vi "TCP_NODELAY.vi"(8 "error in (no error)":errorcluster, 10 "Disable Nagle":bool, 11 "Network Connection in":refnum<k5>) -> (0 "error out":errorcluster, 3 "Network Connection out":refnum<k5>)   [LabVIEW 2013, in "Modbus Library - Advance.lvlib"]
doc: "This VI disables the nagle algorithm on a port."
uses:
  Modbus Library - Advance.lvlib
  wsock32.dll
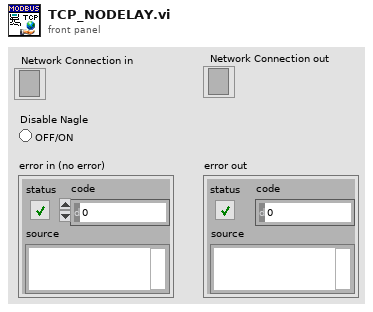
[diagram p1: front panel]
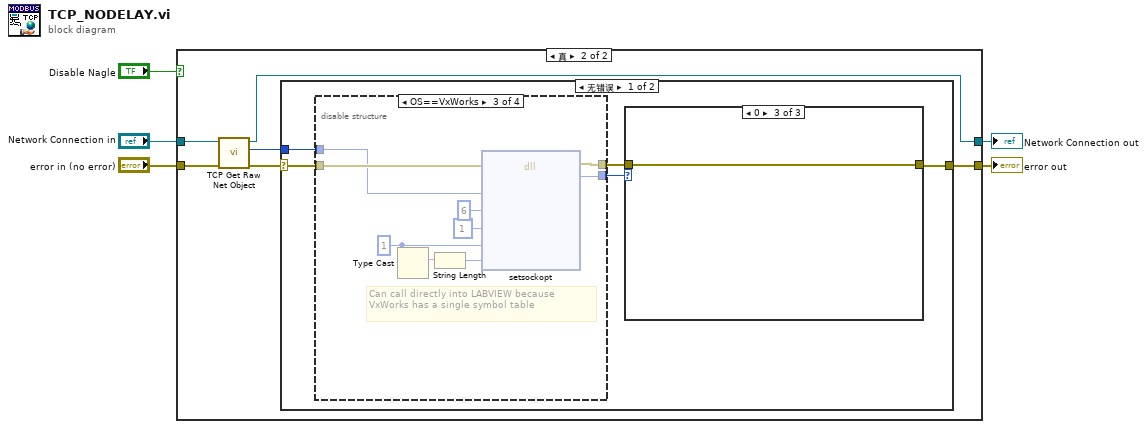
[diagram p0: block diagram]
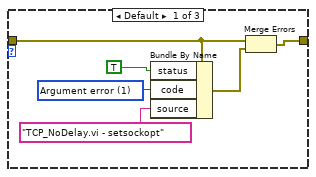
[diagram p3: hidden frame]
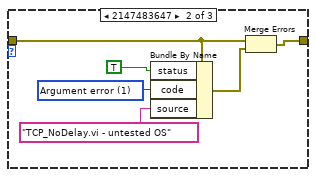
[diagram p4: hidden frame]
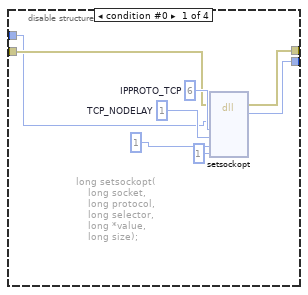
[diagram p5: hidden frame]
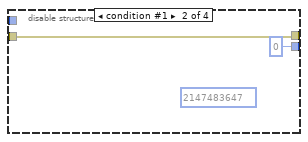
[diagram p6: hidden frame]
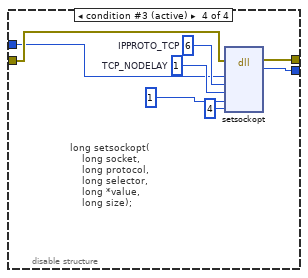
[diagram p7: hidden frame]
diagram:
  n1 = case shown="真" "Disable Nagle" {
    tunnel: "Network Connection in" -> [w7 w13]
    tunnel: [w7 w12] -> w1
    tunnel: "error in (no error)" -> [w6 w11]
    tunnel: [w6 w9] -> w2
    frame False {
    }
    frame True {
      n2 = call <vilib>:"TCP Get Raw Net Object.vi"("error in (no error)"=w11, "connection ID"=w13) -> ("error out"=w10:errorcluster, "raw net object"=w8:u64, "connection ID out"=w12:refnum<k5>)  [unwired: 7 in]
      n3 = case shown="无错误" w10 {
        selector: w10 -> [w18 w59]
        tunnel: [w14 w59] -> w9
        tunnel: w8 -> [w17 _]
        frame No Error {
          n4 = disable-structure shown="OS==VxWorks" {
            disable-tunnel: w18 -> [w36 w41 w45 w52]
            disable-tunnel: w17 -> [w34 _ w42 w51]
            disable-tunnel: [w33 w41 w44 w55] -> w15
            disable-tunnel: [w32 0 w43 w54] -> w16
            frame condition #0 {
              w38 = 1  # TCP_NODELAY
              w37 = 6  # IPPROTO_TCP
              # "long setsockopt(\n    long socket,\n    long protocol,\n    long selector,\n    long *value,\n    long size);"
              n5 = dll-call lib="wsock32.dll" fn="setsockopt" ("Call Library Function")(error in=w36, "socket"=w34, "protocol"=w37, "selector"=w38, "value"=u8 1, "size"=1) -> (error out=w33:errorcluster, w32:i32)  [unwired: 7 in, 1 out]
            }
            frame condition #1 {
              (unwired) 2147483647
            }
            frame condition #2 {
              w48 = 1 ("(char*) &opt")
              # "Can call directly into LABVIEW because\nVxWorks has a single symbol table"
              n6 = Type Cast(x=w48) -> (*(type *) &x=w49:string)  [unwired: 1 in]
              n7 = String Length(string=w49) -> (length=w50:i32)
              n8 = dll-call lib="LabVIEW" fn="setsockopt"(error in=w45, "socket"=w42, "IPPROTO"=6, "option name"=1, "(char*) &opt"=w48, "sizeof(opt)"=w50) -> (error out=w44:errorcluster, "return"=w43:u8)  [unwired: 7 in, 1 out]
            }
            frame condition #3 (active) {
              w57 = 1  # TCP_NODELAY
              w58 = 6  # IPPROTO_TCP
              # "long setsockopt(\n    long socket,\n    long protocol,\n    long selector,\n    long *value,\n    long size);"
              n9 = dll-call lib="wsock32.dll" fn="setsockopt" ("Call Library Function")(error in=w52, "socket"=w51, "protocol"=w58, "selector"=w57, "value"=u8 1, "size"=4) -> (error out=w55:errorcluster, "return type"=w54:i32)  [unwired: 7 in, 1 out]
            }
          }
          n10 = case shown="0" w16 {
            tunnel: [w20 w26 w31] -> w14
            tunnel: w15 -> [w19 w25 w31]
            frame Default {
              w24 = 1 items=["No error", "Argument error", "Memory is full", "Out of zone", "End of file", "File already open", "Generic file I/O error", "File not found", "File permission error", "Disk is full", "Duplicate path", "Too many files open", "System feature not enabled", "Resource file not found", "Cannot add resource", "Resource not found", "Image not found", "Image memory error", "Pen does not exist", "Config type invalid", "Config token not found", "Config parse error", "Config memory error", "Bad external code format", "Bad external code offset", "External code not present", "Null window", "Destroy window error", "Null menu", "Print aborted", "Bad print record", "Print driver error", "Windows error during printing", "Memory error during printing", "Print dialog error", "Generic print error", "Invalid device refnum", "Device not found", "Device parameter error", "Device unit error", "Cannot open device", "Device call aborted", "Generic error", "Cancelled by user", "Object ID too low", "Object ID too high", "Object not in heap", "Unknown heap", "Unknown object (invalid DefProc)", "Unknown object (DefProc not in table)", "Message out of range", "Invalid (null) method", "Unknown message", "Manager call not supported", "Bad address", "Network operation in progress", "Network operation timed out", "Connection is busy", "Network attribute not supported", "Network error", "Address in use", "System out of memory", "Connection aborted", "Connection refused", "Not connected", "Already connected", "Connection closed", "Initialization error (interapplication manager)", "Bad occurrence", "Wait on unbound occurrence handler", "Occurrence queue overflow", "Datalog type conflict", "Unused", "Unrecognized type (interapplication manager)", "Memory corrupt", "Failed to make temporary DLL", "Old CIN version", "Drag socket not found", "Failed to load drop-object", "Failed to register OLE object", "Failed to release OLE object", "Format specifier type mismatch", "Unknown format specifier", "Too few format specifiers", "Too many format specifiers", "Scan failed", "Newer CIN version", "Error converting to variant", "Runtime menu error", "Password tampered", "Variant attribute not found", "Incompatible variant data type", "Event data is not available", "Event Store is not present", "Occurrence is not found", "Event Queue is not created", "Event info is not available", "Refnum passed is NULL", "Error retrieving Class GUID", "Error retrieving CoClass GUID", "Error retrieving TypeLib GUID.", "Bad built application magic bytes.", "Specific driver is different from the specific driver associated with the Logical Name.", "There is no session opened to the class driver.", "Max Error", "MAX - Error with config objects", "MAX - Error loading configuration", "MAX - Group not supported"]
              n11 = Bundle By Name(cluster=w19, "status"=TRUE, "code"=w24, "source"="TCP_NoDelay.vi - setsockopt") -> (w21:errorcluster)
              n12 = Merge Errors(w19, w21) -> (w20:errorcluster)
            }
            frame 2147483647 {
              w30 = 1 items=["No error", "Argument error", "Memory is full", "Out of zone", "End of file", "File already open", "Generic file I/O error", "File not found", "File permission error", "Disk is full", "Duplicate path", "Too many files open", "System feature not enabled", "Resource file not found", "Cannot add resource", "Resource not found", "Image not found", "Image memory error", "Pen does not exist", "Config type invalid", "Config token not found", "Config parse error", "Config memory error", "Bad external code format", "Bad external code offset", "External code not present", "Null window", "Destroy window error", "Null menu", "Print aborted", "Bad print record", "Print driver error", "Windows error during printing", "Memory error during printing", "Print dialog error", "Generic print error", "Invalid device refnum", "Device not found", "Device parameter error", "Device unit error", "Cannot open device", "Device call aborted", "Generic error", "Cancelled by user", "Object ID too low", "Object ID too high", "Object not in heap", "Unknown heap", "Unknown object (invalid DefProc)", "Unknown object (DefProc not in table)", "Message out of range", "Invalid (null) method", "Unknown message", "Manager call not supported", "Bad address", "Network operation in progress", "Network operation timed out", "Connection is busy", "Network attribute not supported", "Network error", "Address in use", "System out of memory", "Connection aborted", "Connection refused", "Not connected", "Already connected", "Connection closed", "Initialization error (interapplication manager)", "Bad occurrence", "Wait on unbound occurrence handler", "Occurrence queue overflow", "Datalog type conflict", "Unused", "Unrecognized type (interapplication manager)", "Memory corrupt", "Failed to make temporary DLL", "Old CIN version", "Drag socket not found", "Failed to load drop-object", "Failed to register OLE object", "Failed to release OLE object", "Format specifier type mismatch", "Unknown format specifier", "Too few format specifiers", "Too many format specifiers", "Scan failed", "Newer CIN version", "Error converting to variant", "Runtime menu error", "Password tampered", "Variant attribute not found", "Incompatible variant data type", "Event data is not available", "Event Store is not present", "Occurrence is not found", "Event Queue is not created", "Event info is not available", "Refnum passed is NULL", "Error retrieving Class GUID", "Error retrieving CoClass GUID", "Error retrieving TypeLib GUID.", "Bad built application magic bytes.", "Specific driver is different from the specific driver associated with the Logical Name.", "There is no session opened to the class driver.", "Max Error", "MAX - Error with config objects", "MAX - Error loading configuration", "MAX - Group not supported"]
              n13 = Bundle By Name(cluster=w25, "status"=TRUE, "code"=w30, "source"="TCP_NoDelay.vi - untested OS") -> (w27:errorcluster)
              n14 = Merge Errors(w25, w27) -> (w26:errorcluster)
            }
            frame 0 {
            }
          }
        }
        frame Error {
        }
      }
    }
  }
  "error out" <- w2
  "Network Connection out" <- w1
